vi "Example2_wrapback.vi"() -> ()   [LabVIEW 2019]
panel:
  out "error out":errorcluster
  in  "error in (no error)":errorcluster
  in  "Partition":i32
  in  "Topic":string="qamData"
  in  "Kafka Broker":string="localhost:9092"
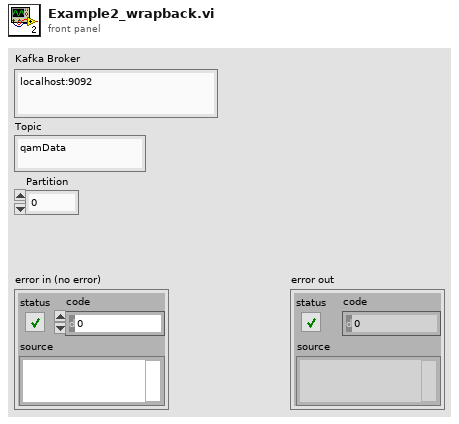
[diagram p1: front panel]
types:
  T1 = typedef "LVKafka.lvlib/KafkaConsumerEvent.ctl" = cluster{"Payload":string, "Key":string, "MsgLen":u64, "Offset":i64, "Time Stamp":i64, "TS Name":string}
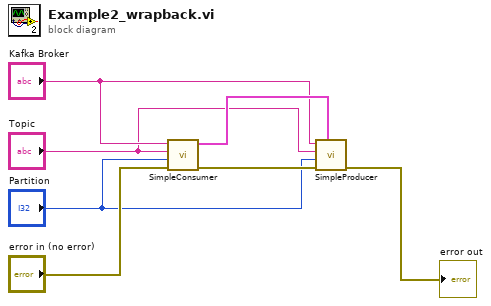
[diagram p0: block diagram]
diagram:
  n1 = call "SimpleConsumer.vi"("error in (no error)"="error in (no error)", "Partition"="Partition", "Topic"="Topic", "Kafka Broker"="Kafka Broker") -> ("error out"=w5:errorcluster, "Events"=w6:T1[])  [unwired: 5 in, 1 out]
  n2 = call "SimpleProducer.vi"("Events"=w6, "error in (no error)"=w5, "Partition"="Partition", "Topic"="Topic", "Kafka Broker"="Kafka Broker") -> ("error out"=→"error out":errorcluster)  [unwired: 6 in]
